vi "Graph Blowup__DV.vi"(8 "error in":errorcluster, 9 "NewRange":T2, 10 "Value":waveform(dbl)[](array[waveform]), 11 "FPButtons":refnum<vi>[](array[refnum])) -> (0 "error out":errorcluster, 3 "数据内容":T3[](array[typedef]) {"峰峰值" format="%#.3f"; "平均值" format="%#.3f"; "最小值" format="%#_3f"; "最大值" format="%#.3f"; "间隔(s)" format="%#.3f"})   [LabVIEW 2012]
doc: "用于相应用户界面对波形的部分截取。根据部分波形来算数据内容。"
uses:
  Waveform Info__DV.ctl
  Channel Info__DV.ctl
  <vilib>/Waveform/WDTOps.llb/WDT Get Waveform Subset DBL.vi
panel:
  in  "通道选择":T1[](array[typedef]) {"type" items=["SC1Mod1/ai0", "SC1Mod2/ai0", "SC1Mod3/ai0", "DSA/ai0", "DSA/ai1"]}
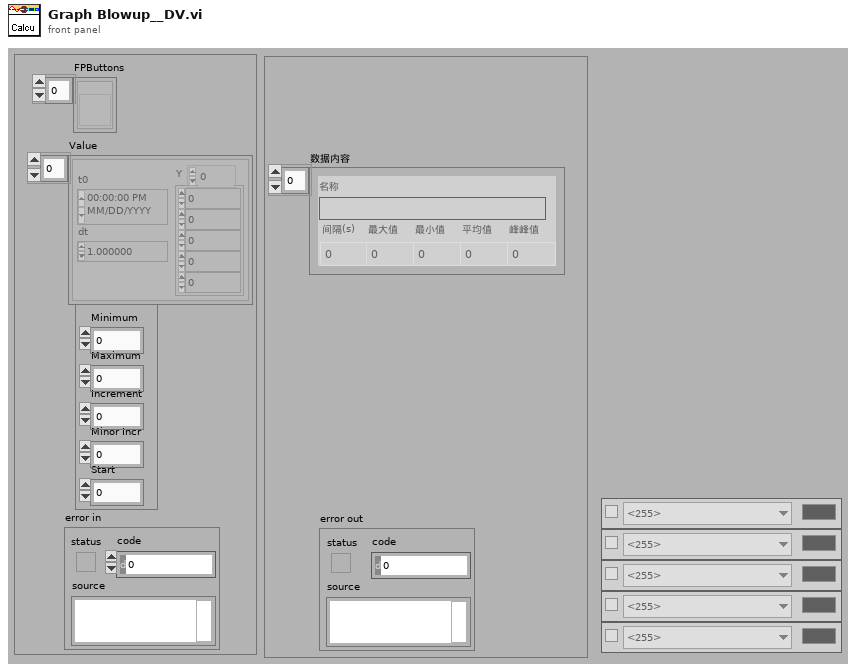
[diagram p1: front panel]
types:
  T1 = typedef "Channel Info__DV.ctl" = cluster{"in use":bool, "color":u32, "type":u16}
  T2 = cluster{"Minimum":dbl, "Maximum":dbl, "Increment":dbl, "Minor Incr":dbl, "Start":dbl}
  T3 = typedef "Waveform Info__DV.ctl" = cluster{"间隔(s)":dbl, "最大值":dbl, "最小值":dbl, "平均值":dbl, "峰峰值":dbl, "名称":string}
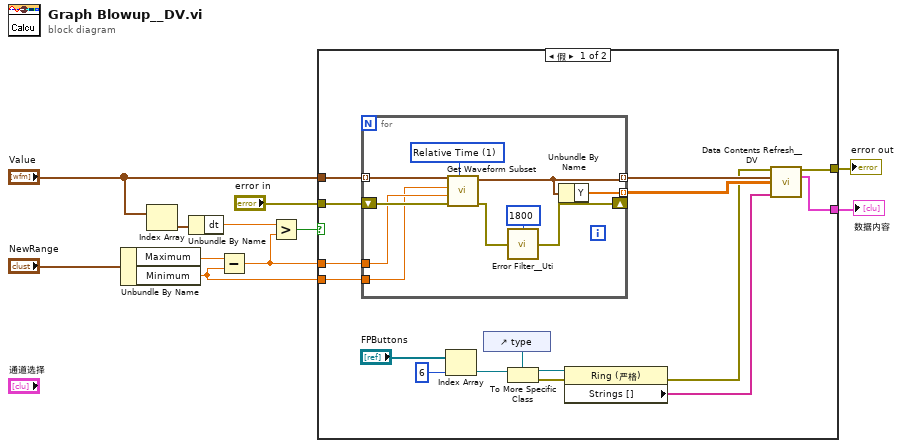
[diagram p0: block diagram]
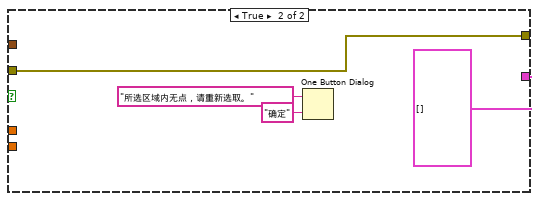
[diagram p2: hidden frame]
diagram:
  n1 = Unbundle By Name("NewRange") -> ("Maximum"=w10:dbl, "Minimum"=w1:dbl)
  n2 = Index Array(array="Value") -> (element=w5:waveform(dbl))  [unwired: 1 in]
  n3 = Unbundle By Name(w5) -> ("dt"=w4:dbl)
  n4 = Subtract(x=w10, y=w1) -> (x-y=w2:dbl)
  n5 = Greater?(x=w4, y=w2) -> (0:w3:bool)
  n6 = case shown="假" w3 {
    tunnel: "Value" -> [w27 _]
    tunnel: "error in" -> [w26 w41]
    tunnel: [w23 w41] -> w8
    tunnel: [w22 T3[] [] ("数据内容")] -> w11
    tunnel: w2 -> [w13 _]
    tunnel: w1 -> [w12 _]
    frame False {
      n7 = for {
        tunnel: w27 -> [w37] mode=indexing
        shift-right: [w30] -> _
        shift-left: w26 -> [w36]
        tunnel: [w35] -> w25 mode=indexing
        tunnel: [w34] -> w24 mode=indexing
        tunnel: w13 -> [w29]
        tunnel: w12 -> [w28]
        w33 = u16 1 items=["Samples", "Relative Time"] ("start/duration format")
        n8 = call-poly <vilib>:"Get Waveform Subset.vi"("start/duration format"=w33, "error in (no error)"=w36, "duration"=w29, "start samples/time"=w28, "waveform in"=w37) -> ("error out"=w31:errorcluster, "waveform out"=w35:waveform(dbl))  [unwired: 1 in, 2 out]
        n9 = call "Error Filter__Uti.vi"("error in"=w31, "error to filter"=1800) -> ("error out"=w30:errorcluster)
        n10 = Unbundle By Name(w35) -> ("Y"=w34:dbl[])
      }
      n11 = Index Array(array="FPButtons", index=6) -> (element=w20:refnum<vi>)
      n12 = control-ref of="type"() -> (w15:refnum<vi>)
      n13 = To More Specific Class(target class=w15, reference=w20) -> (specific class reference=w18:refnum<vi>, error out=w19:errorcluster)  [unwired: 1 in]
      n14 = property class="Ring (严格)"(reference=w18, error in=w19) -> (error out=w16:errorcluster, "Strings []"=w17:string[])  [unwired: 1 out]
      n15 = call "Data Contents Refresh__DV.vi"("error in (no error)"=w16, "Graph Refreshed"=w25, "Data 2DDBL"=w24, "Array"=w17) -> ("error out"=w23:errorcluster, "数据内容"=w22:T3[])  [unwired: 10 in]
    }
    frame True {
      n16 = One Button Dialog(message="所选区域内无点，请重新选取。", button name ("OK")="确定") -> ()  [unwired: 1 out]
    }
  }
  "数据内容" <- w11
  "error out" <- w8
